vi "CalculationProjectionAngleOffset.vi"(6 "Y offset":dbl, 7 "X offset":dbl, 9 "Angle":dbl, 10 "Height":dbl, 11 "Width":dbl) -> (1 "ResultY":dbl, 2 "ResultX":dbl)   [LabVIEW 2016]
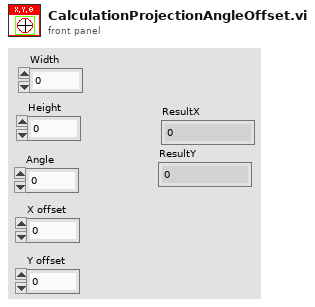
[diagram p1: front panel]
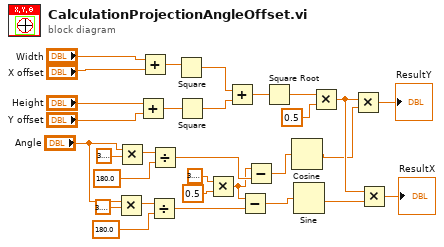
[diagram p0: block diagram]
diagram:
  n1 = Multiply(x="Angle", y=3.141592653589793) -> (x*y=w14:dbl)
  n2 = Multiply(x="Angle", y=3.141592653589793) -> (x*y=w17:dbl)
  n3 = Add(x="Height", y="Y offset") -> (x+y=w19:dbl)
  n4 = Add(x="Width", y="X offset") -> (x+y=w20:dbl)
  n5 = Divide(x=w14, y=180.0) -> (x/y=w5:dbl)
  n6 = Divide(x=w17, y=180.0) -> (x/y=w7:dbl)
  n7 = Square(x=w20) -> (x^2=w26:dbl)
  n8 = Square(x=w19) -> (x^2=w25:dbl)
  n9 = Multiply(x=3.141592653589793, y=0.5) -> (x*y=w6:dbl)
  n10 = Add(x=w26, y=w25) -> (x+y=w24:dbl)
  n11 = Subtract(x=w6, y=w5) -> (x-y=w1:dbl)
  n12 = Subtract(x=w6, y=w7) -> (x-y=w4:dbl)
  n13 = Square Root(x=w24) -> (sqrt(x)=w22:dbl)
  n14 = Cosine(x=w4) -> (cos(x)=w3:dbl)
  n15 = Sine(x=w1) -> (sin(x)=w2:dbl)
  n16 = Multiply(x=w22, y=0.5) -> (x*y=w12:dbl)
  n17 = Multiply(x=w12, y=w3) -> (x*y=→"ResultY":dbl)
  n18 = Multiply(x=w12, y=w2) -> (x*y=→"ResultX":dbl)
